vi "FujiDelta Test.vi"() -> ()   [LabVIEW 2014]
uses:
  ALPHA5 RS485/typedefs/Port Selection Info.ctl
  Common/Delta Robot Kinematics/Delta Robot Param.ctl
  Delta Robot/Fuji Delta Robot.lvclass/Fuji Delta Robot.ctl
  ALPHA5 RS485/Classes/FujiMotor/FujiMotor.lvclass
  Common/Delta Robot Kinematics/Delta Robot Kinematics.lvclass
  Delta Robot/Fuji Delta Robot.lvclass
  ALPHA5 RS485/ALPHA5 RS485.lvlib
panel:
  in  "auto time":u32=2000
  in  "auto run":bool
  out "end":bool
  in  "index":i32(ring) items=["X", "Y", "Z"]
  out "Waveform Chart 4":cluster{"Numeric":dbl, "X":dbl, "Numeric":dbl}(graph)
  out "sensed joints":dbl[](array[numeric])
  in  "Set Pos":bool
  in  "Position Cmd":cluster{"X":dbl, "Y":dbl, "Z":dbl} {"Z" scale=-0.8..-0.5; "Y" scale=-0.2..0.2; "X" scale=-0.2..0.2}
  out "Waveform Chart 3":cluster{"Slide":dbl, "ENC Pos":i32}(graph)
  out "Waveform Chart 2":cluster{"Slide":dbl, "ENC Pos":i32}(graph)
  in  "ON/OFF":bool[](array[boolean])=[FALSE, FALSE, FALSE]
  in  "Joints":dbl[](array[slide])=[0.0, 0.0, 0.0]
  in  "stop":bool
  in  "Inst Vel":i32=20000
  out "Waveform Chart":cluster{"Slide":dbl, "ENC Pos":i32}(graph)
  in  "Port Selection Info In":T1={"Port Name"="COM5", "Amplifier Num"=1, "Baud Rate"=38400, "Char Formation"=enum."0"} {"Baud Rate" items=["38400"=38400, "19200"=19200, "9600"=9600, "115200"=0]; "Amplifier Num" max=31}
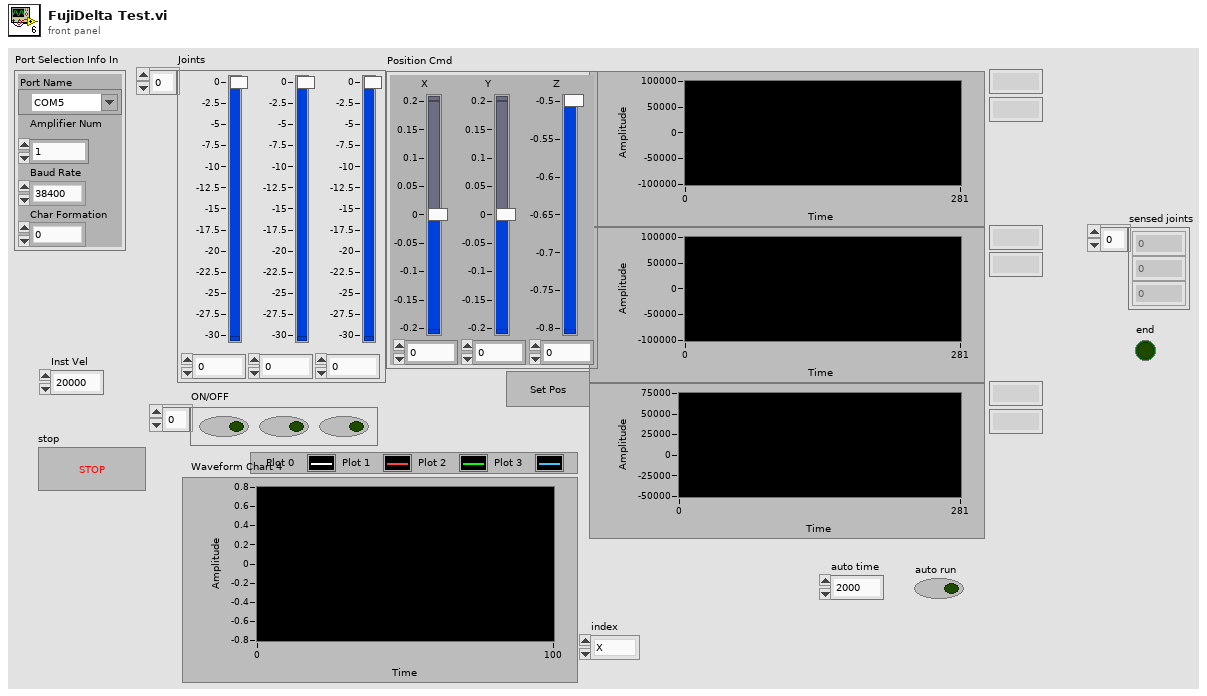
[diagram p1: front panel]
types:
  T1 = typedef "ALPHA5 RS485.lvlib/Port Selection Info.ctl" = cluster{"Port Name":refnum<visa-resource-name>, "Amplifier Num":u8, "Baud Rate":u32, "Char Formation":enum16{"0", "1", "2", "3", "4", "5"}}
  T2 = typedef "Delta Robot Kinematics.lvclass/Delta Robot Param.ctl" = cluster{"f":dbl, "e":dbl, "rf":dbl, "re":dbl}
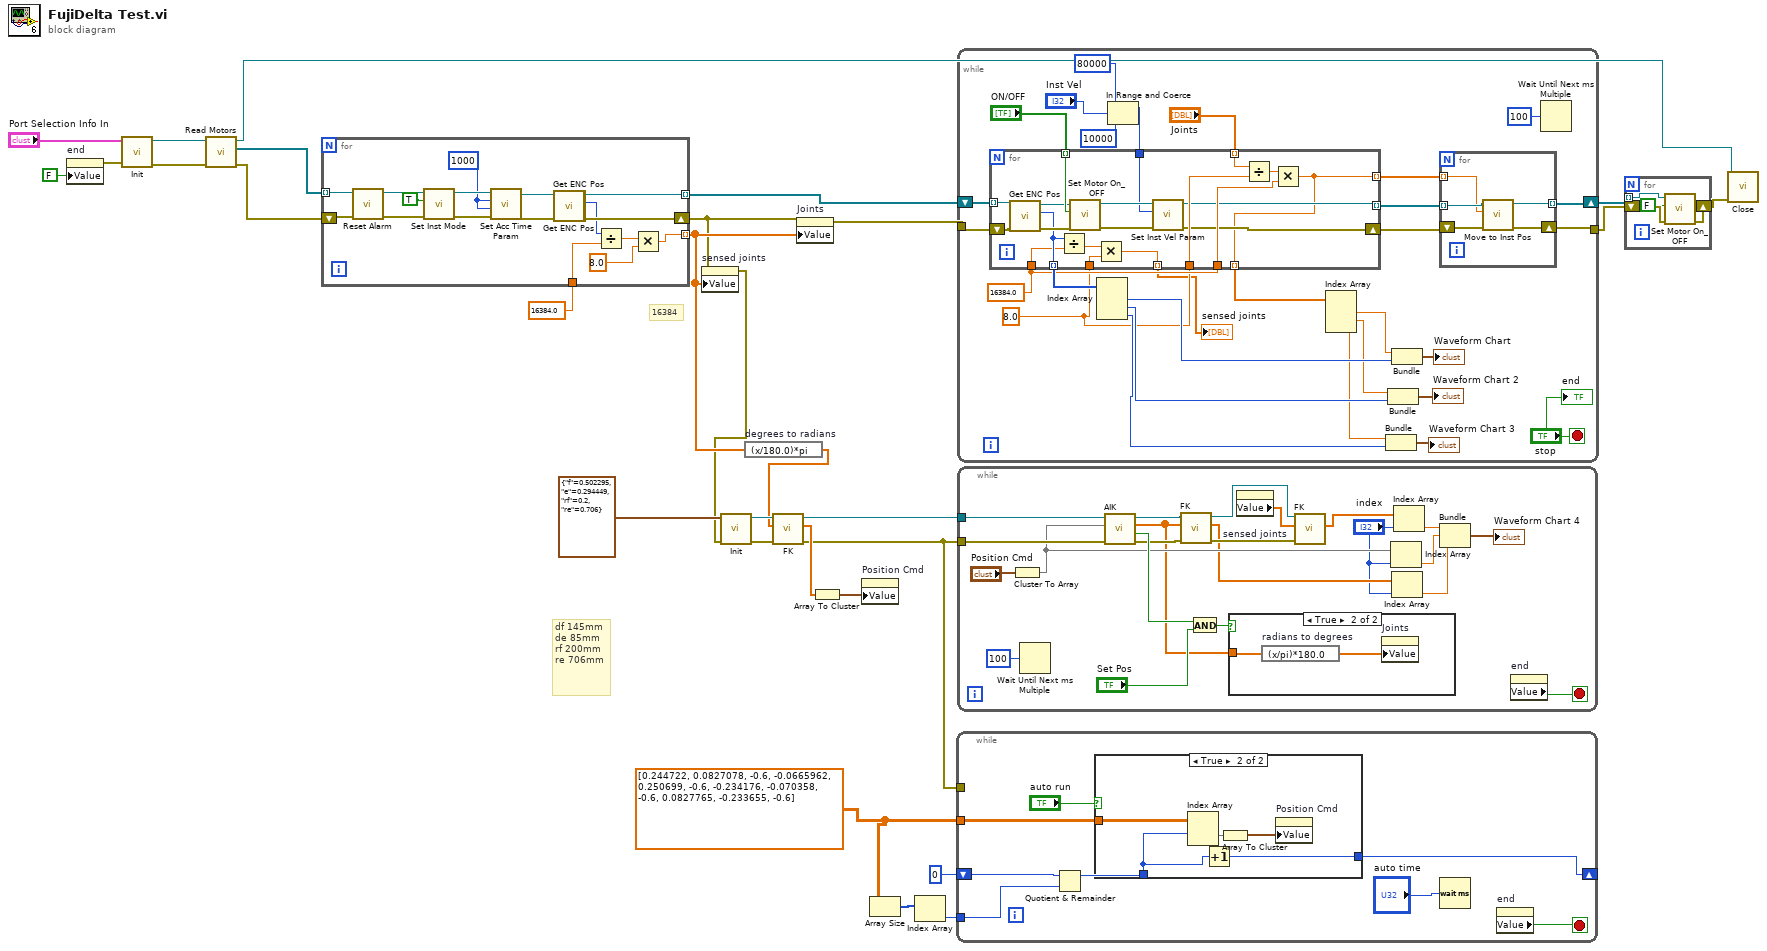
[diagram p0: block diagram]
diagram:
  w3 = dbl[][] [[0.244722, 0.0827078, -0.6], [-0.0665962, 0.250699, -0.6], [-0.234176, -0.070358, -0.6], [0.0827765, -0.233655, -0.6]]
  # "df 145mm\nde 85mm\nrf 200mm \nre 706mm"
  # "16384"
  n1 = property on="end" class="Bool (strict)"("Value"=FALSE ("end")) -> (error out=w7:errorcluster)  [unwired: 2 in, 1 out]
  n2 = call "Init.vi"("error in (no error)"=w7, "Port Selection Info In"="Port Selection Info In") -> ("error out"=w27:errorcluster, "Fuji Delta out"=w28:refnum<class "Fuji Delta Robot.lvclass">)  [unwired: 8 in]
  n3 = call "Read Motors.vi"("error in (no error)"=w27, "Fuji Delta Robot in"=w28) -> ("error out"=w21:errorcluster, "Motors"=w20:refnum<class "FujiMotor.lvclass">[], "Fuji Delta Robot out"=w26:refnum<class "Fuji Delta Robot.lvclass">)  [unwired: 7 in]
  n4 = for {
    tunnel: [w41] -> w22 mode=indexing
    shift-right: [w39] -> w9
    shift-left: w21 -> [w36]
    tunnel: w20 -> [w35] mode=indexing
    tunnel: [w30] -> w10 mode=indexing
    tunnel: 16384.0 ("y") -> [w33]
    w43 = 1000 ("ACC Time")
    n5 = call "Reset Alarm.vi"("error in (no error)"=w36, "FujiMotor in"=w35) -> ("error out"=w37:errorcluster, "FujiMotor out"=w38:refnum<class "FujiMotor.lvclass">)  [unwired: 8 in]
    n6 = call "Set Inst Mode.vi"("error in (no error)"=w37, "ABS/INC"=TRUE, "FujiMotor in"=w38) -> ("error out"=w44:errorcluster, "FujiMotor out"=w45:refnum<class "FujiMotor.lvclass">)  [unwired: 7 in]
    n7 = call "Set Acc Time Param.vi"("error in (no error)"=w44, "DEC Time"=w43, "ACC Time"=w43, "FujiMotor in"=w45) -> ("error out"=w40:errorcluster, "FujiMotor out"=w42:refnum<class "FujiMotor.lvclass">)  [unwired: 6 in]
    n8 = call "Get ENC Pos.vi"("FujiMotor in"=w42) -> ()  [unwired: 8 in, 3 out]
    n9 = call "Get ENC Pos.vi"("error in (no error)"=w40, "FujiMotor in"=w42) -> ("error out"=w39:errorcluster, "ENC Pos"=w34:i32, "FujiMotor out"=w41:refnum<class "FujiMotor.lvclass">)  [unwired: 7 in]
    n10 = Divide(x=w34, y=w33) -> (x/y=w32:dbl)
    n11 = Multiply(x=w32, y=8.0) -> (x*y=w30:dbl)
  }
  n12 = property on="sensed joints" class="Arr (strict)"(error in=w9, "Value"=w10) -> (error out=w8:errorcluster)  [unwired: 1 in, 1 out]
  n13 = call "Init.vi"("error in (no error)"=w8, "Delta Param"=T2 {"f"=0.502295, "e"=0.294449, "rf"=0.2, "re"=0.706}) -> ("error out"=w16:errorcluster, "Delta Robot Kin"=w15:refnum<class "Delta Robot Kinematics.lvclass">)  [unwired: 8 in]
  n14 = expression code="(x/180.0)*pi" "degrees to radians"(w10) -> (w13:dbl[])
  n15 = call-dynamic "FK.vi"("error in (no error)"=w16, "joints"=w13, "Delta Robot Kinematics in"=w15) -> ("error out"=w5:errorcluster, "p"=w12:dbl[], "Delta Robot Kinematics out"=w14:refnum<class "Delta Robot Kinematics.lvclass">)  [unwired: 5 in, 1 out]
  n16 = property on="Joints" class="Arr (strict)"(error in=w9, "Value"=w10) -> (error out=w19:errorcluster)  [unwired: 1 in, 1 out]
  n17 = Array To Cluster(array=w12) -> (cluster=w11:cluster{"p[0]":dbl, "p[1]":dbl, "p[2]":dbl})
  n18 = property on="Position Cmd" class="Clust (strict)"("Value"=w11) -> ()  [unwired: 2 in, 2 out]
  n19 = Array Size(array=w3) -> (size(s)=w2:i32[])
  n20 = Index Array(array=w2) -> (element=w1:i32)  [unwired: 1 in]
  n21 = while {
    tunnel: w5 -> [_]
    tunnel: w3 -> [w50]
    shift-right: [w48] -> _
    shift-left: 0 -> [w52]
    tunnel: w1 -> [w47]
    stop <- w53 stop-if-true
    n22 = Quotient & Remainder(x=w52, y=w47) -> (x-y*floor(x/y)=w49:i32)  [unwired: 1 out]
    n23 = case shown="True" "auto run" {
      tunnel: w50 -> [_ w60]
      tunnel: w49 -> [w55 w57]
      tunnel: [w55 w56] -> w48
      frame False {
      }
      frame True {
        n24 = Index Array(array=w60, index (row)=w57) -> (element=w59:dbl[])  [unwired: 1 in]
        n25 = Increment(x=w57) -> (x+1=w56:i32)
        n26 = Array To Cluster(array=w59) -> (cluster=w58:cluster{"[0]":dbl, "[1]":dbl, "[2]":dbl})
        n27 = property on="Position Cmd" class="Clust (strict)"("Value"=w58) -> ()  [unwired: 2 in, 2 out]
      }
    }
    n28 = Wait (ms)(milliseconds to wait="auto time") -> ()  [unwired: 1 out]
    n29 = property on="end" class="Bool (strict)"() -> ("Value"=w53:bool)  [unwired: 2 in, 2 out]
  }
  n30 = while {
    tunnel: w19 -> [w88]
    tunnel: [w67] -> w24
    shift-right: [w69] -> w25
    shift-left: w22 -> [w89]
    stop <- "stop" stop-if-true
    w73 = 8.0 ("y")
    w74 = 16384.0 ("y")
    n31 = In Range and Coerce(upper limit=80000, x="Inst Vel", lower limit=10000) -> (coerced(x)=w61:i32)  [unwired: 1 out]
    n32 = for {
      tunnel: "ON/OFF" -> [w114] mode=indexing
      tunnel: w61 -> [w111]
      tunnel: [w97] -> w70 mode=indexing
      tunnel: w89 -> [w110] mode=indexing
      tunnel: [w95] -> w83 mode=indexing
      tunnel: [w104] -> w84 mode=indexing
      shift-right: [w96] -> w68
      shift-left: w88 -> [w109]
      tunnel: "Joints" -> [w106] mode=indexing
      tunnel: w74 -> [w103]
      tunnel: w74 -> [w102]
      tunnel: w73 -> [w100]
      tunnel: w73 -> [w99]
      tunnel: [w98] -> w72 mode=indexing
      tunnel: [w95] -> w66 mode=indexing
      n33 = call "Get ENC Pos.vi"("error in (no error)"=w109, "FujiMotor in"=w110) -> ("error out"=w108:errorcluster, "ENC Pos"=w104:i32, "FujiMotor out"=w107:refnum<class "FujiMotor.lvclass">)  [unwired: 7 in]
      n34 = Divide(x=w104, y=w103) -> (x/y=w101:dbl)
      n35 = call "Set Motor On_OFF.vi"("error in (no error)"=w108, "ON/OFF"=w114, "FujiMotor in"=w107) -> ("error out"=w113:errorcluster, "FujiMotor out"=w112:refnum<class "FujiMotor.lvclass">)  [unwired: 7 in]
      n36 = Multiply(x=w101, y=w100) -> (x*y=w98:dbl)
      n37 = call "Set Inst Vel Param.vi"("error in (no error)"=w113, "Inst Vel"=w111, "FujiMotor in"=w112) -> ("error out"=w96:errorcluster, "FujiMotor out"=w97:refnum<class "FujiMotor.lvclass">)  [unwired: 7 in]
      n38 = Divide(x=w106, y=w99) -> (x/y=w105:dbl)
      n39 = Multiply(x=w105, y=w102) -> (x*y=w95:dbl)
    }
    "sensed joints" <- w72
    n40 = Index Array(array=w84) -> (element #1=w81:i32, element #2=w79:i32, element #3=w77:i32)  [unwired: 3 in]
    n41 = Index Array(array=w83) -> (element #1=w82:dbl, element #2=w80:dbl, element #3=w78:dbl)  [unwired: 3 in]
    n42 = Bundle(w78, "ENC Pos"=w77) -> (→"Waveform Chart 3":cluster{dbl, "ENC Pos":i32})  [unwired: 1 in]
    n43 = Bundle(w80, "ENC Pos"=w79) -> (→"Waveform Chart 2":cluster{dbl, "ENC Pos":i32})  [unwired: 1 in]
    n44 = Bundle(w82, "ENC Pos"=w81) -> (→"Waveform Chart":cluster{dbl, "ENC Pos":i32})  [unwired: 1 in]
    n45 = for {
      tunnel: w70 -> [w94] mode=indexing
      tunnel: [w93] -> w69 mode=indexing
      shift-right: [w91] -> w67
      shift-left: w68 -> [w92]
      tunnel: w66 -> [w90] mode=indexing
      n46 = call "Move to Inst Pos.vi"("error in (no error)"=w92, "Inst Pos"=w90, "FujiMotor in"=w94) -> ("error out"=w91:errorcluster, "FujiMotor out"=w93:refnum<class "FujiMotor.lvclass">)  [unwired: 7 in]
    }
    n47 = Wait Until Next ms Multiple(millisecond multiple=u32 100) -> ()  [unwired: 1 out]
    "end" <- "stop"
  }
  n48 = while {
    tunnel: w14 -> [w136]
    tunnel: w5 -> [w135]
    stop <- w116 stop-if-true
    n49 = Cluster To Array(cluster="Position Cmd") -> (array=w125:dbl[])
    n50 = Wait Until Next ms Multiple(millisecond multiple=u32 100) -> ()  [unwired: 1 out]
    n51 = call-dynamic "AIK.vi"("error in (no error)"=w135, "p"=w125, "Delta Robot Kinematics in"=w136) -> ("error out"=w128:errorcluster, "exist"=w131:bool, "joints"=w117:dbl[], "Delta Robot Kinematics out"=w129:refnum<class "Delta Robot Kinematics.lvclass">)  [unwired: 5 in]
    n52 = call-dynamic "FK.vi"("error in (no error)"=w128, "joints"=w117, "Delta Robot Kinematics in"=w129) -> ("error out"=w127:errorcluster, "p"=w124:dbl[], "Delta Robot Kinematics out"=w126:refnum<class "Delta Robot Kinematics.lvclass">)  [unwired: 5 in, 1 out]
    n53 = And(x=w131, y="Set Pos") -> (x .and. y?=w132:bool)
    n54 = case shown="True" w132 {
      tunnel: w117 -> [_ w138]
      frame False {
      }
      frame True {
        n55 = expression code="(x/pi)*180.0" "radians to degrees"(w138) -> (w137:dbl[])
        n56 = property on="Joints" class="Arr (strict)"("Value"=w137) -> ()  [unwired: 2 in, 2 out]
      }
    }
    n57 = property on="sensed joints" class="Arr (strict)"() -> ("Value"=w133:dbl[])  [unwired: 2 in, 2 out]
    n58 = call-dynamic "FK.vi"("error in (no error)"=w127, "joints"=w133, "Delta Robot Kinematics in"=w126) -> ("p"=w123:dbl[])  [unwired: 5 in, 3 out]
    n59 = Index Array(array=w125, index="index") -> (element=w120:dbl)
    n60 = Index Array(array=w124, index="index") -> (element=w119:dbl)
    n61 = Index Array(array=w123, index="index") -> (element=w121:dbl)
    n62 = Bundle("Numeric"=w121, "X"=w120, "Numeric"=w119) -> (→"Waveform Chart 4":cluster{"Numeric":dbl, "X":dbl, "Numeric":dbl})  [unwired: 1 in]
    n63 = property on="end" class="Bool (strict)"() -> ("Value"=w116:bool)  [unwired: 2 in, 2 out]
  }
  n64 = for {
    tunnel: w25 -> [w142] mode=indexing
    shift-right: [w140] -> w23
    shift-left: w24 -> [w141]
    n65 = call "Set Motor On_OFF.vi"("error in (no error)"=w141, "ON/OFF"=FALSE, "FujiMotor in"=w142) -> ("error out"=w140:errorcluster)  [unwired: 7 in, 1 out]
  }
  n66 = call "Close.vi"("error in (no error)"=w23, "Fuji Delta in"=w26) -> ()  [unwired: 9 in, 1 out]
